vi "CMI Sync V3 Set Fixed Session Parameters.vi"(8 "error in":errorcluster, 11 "session in":T1={"VISA"="", "baud rate [bd/s]"=115200, "source"=enum."Auto", "hv range"=enum."1kV", "fsrc is fixed"=FALSE, "fsrc [Hz]"=10000000.0, "freq integ [s]"=1.0, "freq filter"=5, "trig level"=enum."TTL 5V", "chn1 mode"=enum."Source divider", "chn1 level"=enum."Positive 5V", "chn2 mode"=enum."Source divider", "chn2 level"=enum."Positive 5V", "chn2 div"=1, "chn3 mode"=enum."Chn 1 Active", "chn3 level"=enum."Positive 5V"} {"chn2 div" min=1 max=100000000 step=1; "fsrc [Hz]" format="%_8p"}) -> (0 "error out":errorcluster, 3 "session out":T1={"VISA"="", "baud rate [bd/s]"=115200, "source"=enum."Auto", "hv range"=enum."1kV", "fsrc is fixed"=FALSE, "fsrc [Hz]"=10000000.0, "freq integ [s]"=1.0, "freq filter"=5, "trig level"=enum."TTL 5V", "chn1 mode"=enum."Source divider", "chn1 level"=enum."Positive 5V", "chn2 mode"=enum."Source divider", "chn2 level"=enum."Positive 5V", "chn2 div"=1, "chn3 mode"=enum."Chn 1 Active", "chn3 level"=enum."Positive 5V"} {"chn2 div" min=1 max=100000000 step=1; "fsrc [Hz]" format="%_8p"})   [LabVIEW 2020, in "AWG.lvlib" / "CMI Sync Unit V3.lvlib"]
doc: "This is top level VI that will setup unit using parameters defined in session which comes e.g. from Panel.vi. This is intended to be called by e.g. TWM to set whole batch of parameters that are not normally changed after initialization."
uses:
  CMI Sync Unit V3.lvlib
  CMI Sync V3 session.ctl
  Configure/CMI Sync V3 Reference Clock Source.ctl
  Configure/CMI Sync V3 HV input Range.ctl
  Configure/CMI Sync V3 Trigger Input Level.ctl
  Configure/CMI Sync V3 Channel 1 Mode.ctl
  Configure/CMI Sync V3 Channel Output Levels.ctl
  Configure/CMI Sync V3 Channel 2 Mode.ctl
  Configure/CMI Sync V3 Channel 3 Mode.ctl
  Configure/CMI Sync V3 Trigger Mode.ctl
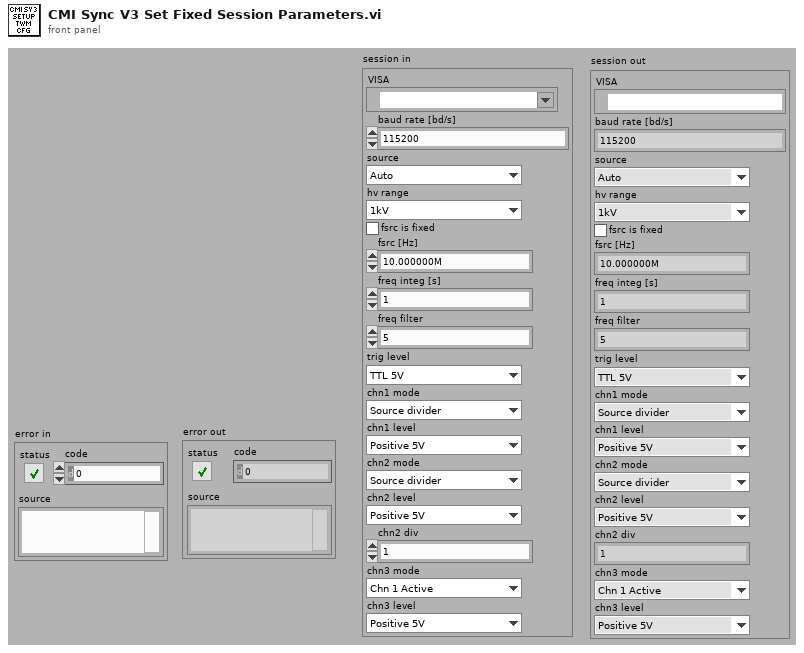
[diagram p1: front panel]
types:
  T1 = typedef "AWG.lvlib/CMI Sync Unit V3.lvlib/CMI Sync V3 session.ctl" = cluster{"VISA":refnum<visa-resource-name>, "baud rate [bd/s]":i32, "source":T2, "hv range":T3, "fsrc is fixed":bool, "fsrc [Hz]":dbl, "freq integ [s]":dbl, "freq filter":i32, "trig level":T4, "chn1 mode":T5, "chn1 level":T6, "chn2 mode":T7, "chn2 level":T6, "chn2 div":i32, "chn3 mode":T8, "chn3 level":T6}
  T2 = typedef "AWG.lvlib/CMI Sync Unit V3.lvlib/CMI Sync V3 Reference Clock Source.ctl" = enum16{"Auto", "Internal", "Logic", "Sine", "HV"}
  T3 = typedef "AWG.lvlib/CMI Sync Unit V3.lvlib/CMI Sync V3 HV input Range.ctl" = enum16{"10V", "60V", "250V", "1kV"}
  T4 = typedef "AWG.lvlib/CMI Sync Unit V3.lvlib/CMI Sync V3 Trigger Input Level.ctl" = enum16{"LVCMOS 3V3", "TTL 5V"}
  T5 = typedef "AWG.lvlib/CMI Sync Unit V3.lvlib/CMI Sync V3 Channel 1 Mode.ctl" = enum16{"Source divider", "DDS absolute", "DDS ratio", "DDS ratio M/N"}
  T6 = typedef "AWG.lvlib/CMI Sync Unit V3.lvlib/CMI Sync V3 Channel Output Levels.ctl" = enum16{"Positive 3V3", "Negative 3V3", "Positive 5V", "Negative 5V"}
  T7 = typedef "AWG.lvlib/CMI Sync Unit V3.lvlib/CMI Sync V3 Channel 2 Mode.ctl" = enum16{"Source divider", "Chn 1 divide"}
  T8 = typedef "AWG.lvlib/CMI Sync Unit V3.lvlib/CMI Sync V3 Channel 3 Mode.ctl" = enum16{"Chn 1 Active", "Chn 2 Active", "Chn 1 Trigger", "Chn 2 Trigger", "Gate", "PPS", "10MHz"}
  T9 = typedef "AWG.lvlib/CMI Sync Unit V3.lvlib/CMI Sync V3 Trigger Mode.ctl" = enum16{"Hold", "Auto (continuous)", "Gate positive", "Gate negative", "Rising edge", "Falling edge", "Bus (*TRG)", "Manual (button)"}
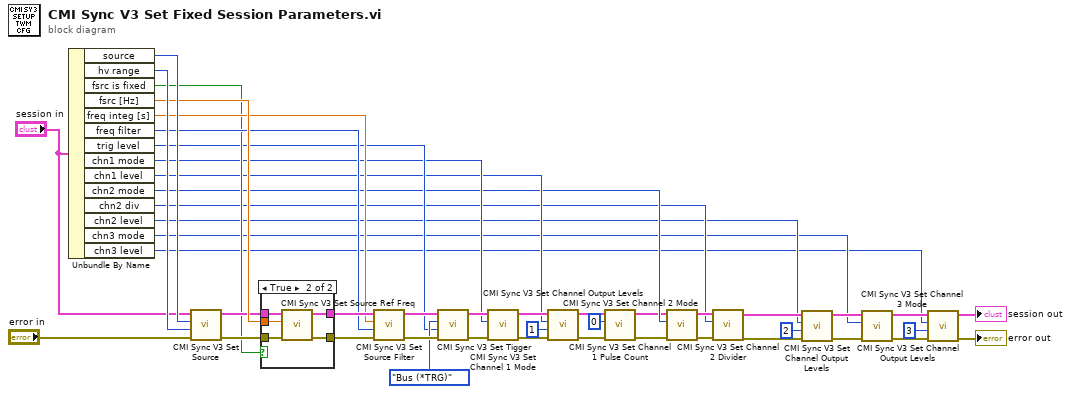
[diagram p0: block diagram]
diagram:
  n1 = Unbundle By Name("session in") -> ("source"=w44:T2, "hv range"=w43:T3, "fsrc is fixed"=w34:bool, "fsrc [Hz]"=w41:dbl, "freq integ [s]"=w36:dbl, "freq filter"=w35:i32, "trig level"=w30:T4, "chn1 mode"=w27:T5, "chn1 level"=w24:T6, "chn2 mode"=w22:T7, "chn2 div"=w19:i32, "chn2 level"=w15:T6, "chn3 mode"=w12:T8, "chn3 level"=w8:T6)
  n2 = call "CMI Sync V3 Set Source.vi"("error in"="error in", "HV range (1kV)"=w43, "Source (Internal)"=w44, "session in"="session in") -> ("error out"=w39:errorcluster, "session out"=w40:T1)  [unwired: 6 in]
  n3 = case shown="True" w34 {
    tunnel: w41 -> [_ w52]
    tunnel: w40 -> [w47 w51]
    tunnel: w39 -> [w46 w50]
    tunnel: [w46 w49] -> w38
    tunnel: [w47 w48] -> w37
    frame False {
    }
    frame True {
      n4 = call "CMI Sync V3 Set Source Ref Freq.vi"("error in"=w50, "Expected reference frequency [Hz]"=w52, "session in"=w51) -> ("error out"=w49:errorcluster, "session out"=w48:T1)  [unwired: 7 in]
    }
  }
  n5 = call "CMI Sync V3 Set Source Filter.vi"("error in"=w38, "Filter cycles (10)"=w35, "Integration time [s]"=w36, "session in"=w37) -> ("error out"=w33:errorcluster, "session out"=w32:T1)  [unwired: 6 in]
  n6 = call "CMI Sync V3 Set Tigger.vi"("error in"=w33, "Trigger input logic (5V)"=w30, "Trigger mode (Auto)"=CMI_Sync_V3_Trigger_Mode."Bus (*TRG)", "session in"=w32) -> ("error out"=w29:errorcluster, "session out"=w28:T1)  [unwired: 6 in]
  n7 = call "CMI Sync V3 Set Channel 1 Mode.vi"("error in"=w29, "Channel 1 mode (DIV)"=w27, "session in"=w28) -> ("error out"=w26:errorcluster, "session out"=w25:T1)  [unwired: 7 in]
  n8 = call "CMI Sync V3 Set Channel Output Levels.vi"("error in"=w26, "Channel index (1)"=1, "Output levels (pos 5V)"=w24, "session in"=w25) -> ("error out"=w5:errorcluster, "session out"=w4:T1)  [unwired: 6 in]
  n9 = call "CMI Sync V3 Set Channel 1 Pulse Count.vi"("error in"=w5, "Pulse count (0: infinite)"=0, "session in"=w4) -> ("error out"=w2:errorcluster, "session out"=w3:T1)  [unwired: 7 in]
  n10 = call "CMI Sync V3 Set Channel 2 Mode.vi"("error in"=w2, "Channel 2 mode (DIV)"=w22, "session in"=w3) -> ("error out"=w21:errorcluster, "session out"=w20:T1)  [unwired: 7 in]
  n11 = call "CMI Sync V3 Set Channel 2 Divider.vi"("error in"=w21, "Divider (10)"=w19, "session in"=w20) -> ("error out"=w17:errorcluster, "session out"=w16:T1)  [unwired: 7 in]
  n12 = call "CMI Sync V3 Set Channel Output Levels.vi"("error in"=w17, "Channel index (1)"=2, "Output levels (pos 5V)"=w15, "session in"=w16) -> ("error out"=w14:errorcluster, "session out"=w13:T1)  [unwired: 6 in]
  n13 = call "CMI Sync V3 Set Channel 3 Mode.vi"("error in"=w14, "Channel 3 mode (10 MHz)"=w12, "session in"=w13) -> ("error out"=w10:errorcluster, "session out"=w9:T1)  [unwired: 7 in]
  n14 = call "CMI Sync V3 Set Channel Output Levels.vi"("error in"=w10, "Channel index (1)"=3, "Output levels (pos 5V)"=w8, "session in"=w9) -> ("error out"=→"error out":errorcluster, "session out"=→"session out":T1)  [unwired: 6 in]
